vi "Set LVLIBP Path.vi"(10 "LVLIBP Path":path, 11 "LVLIBP Parser in":refnum<class "LVLIBP Parser.lvclass">) -> (3 "LVLIBP Parser out":refnum<class "LVLIBP Parser.lvclass">)   [LabVIEW 2019, in "LVLIBP CD XML Updater.lvlib" / "LVLIBP Parser.lvclass"]
uses:
  LVLIBP Parser.lvclass
  LVLIBP Parser.lvclass/LVLIBP Parser.ctl
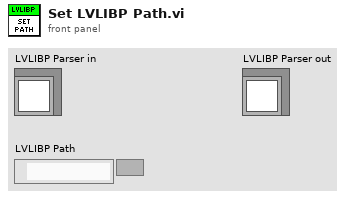
[diagram p1: front panel]
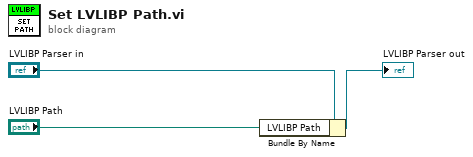
[diagram p0: block diagram]
diagram:
  n1 = Bundle By Name(cluster="LVLIBP Parser in", "LVLIBP Path"="LVLIBP Path") -> (→"LVLIBP Parser out":refnum<class "LVLIBP Parser.lvclass">)
